vi "Level Out S&THx.vi"() -> ()   [LabVIEW 2017]
panel:
  out "Level Out":dbl
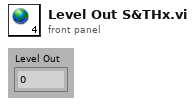
[diagram p1: front panel]
diagram:
